vi "scan_to_position.vi"(4 "VISA resource name":refnum<visa-resource-name>, 6 "Direction to Move":string(combo), 8 "Pixel Size (mm)":string) -> ()   [LabVIEW 2017]
panel:
  in  "Wait before read (0ms)":u32
  in  "Bytes to read (100)":u32=100
  out "Returned string":string
  in  "error in (no error) 2":errorcluster
  out "Command":string
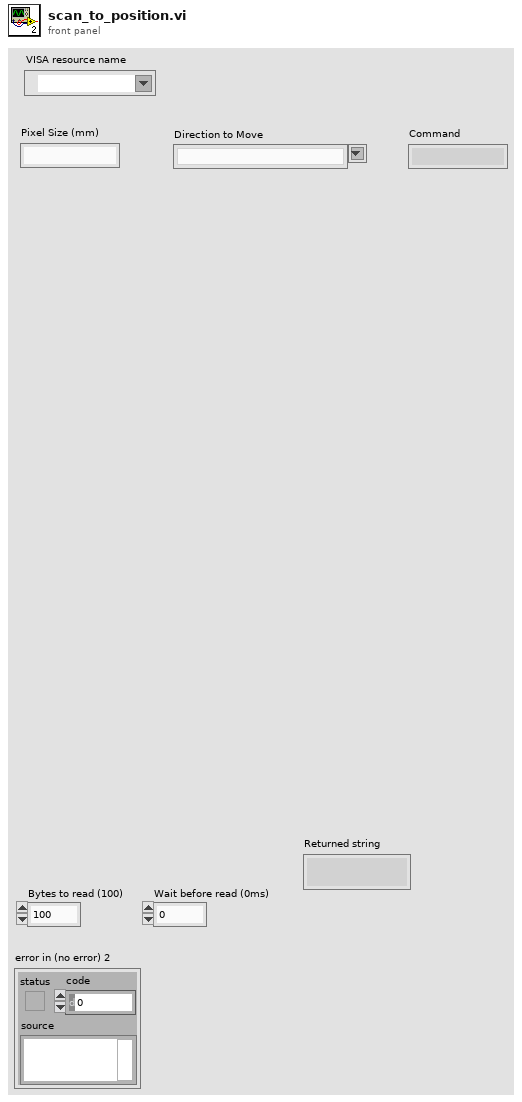
[diagram p1: front panel]
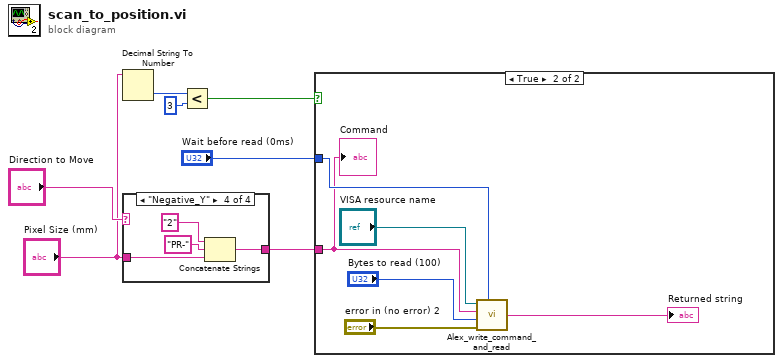
[diagram p0: block diagram]
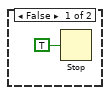
[diagram p2: hidden frame]
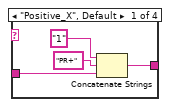
[diagram p3: hidden frame]
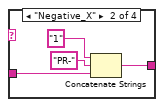
[diagram p4: hidden frame]
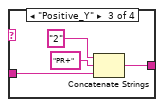
[diagram p5: hidden frame]
diagram:
  n1 = Decimal String To Number(string="Pixel Size (mm)") -> (number=w4:i32)  [unwired: 2 in, 1 out]
  n2 = case shown="\"Negative_Y\"" "Direction to Move" {
    tunnel: [w11 w13 w17 w21] -> w5
    tunnel: "Pixel Size (mm)" -> [w8 w12 w16 w20]
    frame "Positive_X", Default {
      n3 = Concatenate Strings("1", "PR+", w8) -> (w11:string)
    }
    frame "Negative_X" {
      n4 = Concatenate Strings("1", "PR-", w12) -> (w13:string)
    }
    frame "Positive_Y" {
      n5 = Concatenate Strings("2", "PR+", w16) -> (w17:string)
    }
    frame "Negative_Y" {
      n6 = Concatenate Strings("2", "PR-", w20) -> (w21:string)
    }
  }
  n7 = Less?(x=w4, y=3) -> (x < y?=w2:bool)
  n8 = case shown="True" w2 {
    tunnel: "Wait before read (0ms)" -> [_ w28]
    tunnel: w5 -> [_ w26]
    frame False {
      n9 = Stop(stop? (T)=TRUE) -> ()
    }
    frame True {
      n10 = call "Alex_write_command_and_read.vi"("VISA resource name"="VISA resource name", "Wait before read (0ms)"=w28, "Command"=w26, "Bytes to read (100)"="Bytes to read (100)", "error in (no error)"="error in (no error) 2") -> ("Returned string"=→"Returned string":string)  [unwired: 3 in]
      "Command" <- w26
    }
  }
